vi "UI.vi"() -> ()   [LabVIEW 2016]
uses:
  interface_class/interface.lvclass
  <vilib>/Utility/miscctls.llb/LVPointTypeDef.ctl
  <vilib>/picture/picture.llb/imagedata.ctl
  MBinteractive_class/MBinteractive.lvclass
  tcp_work_class/tcp_work.lvclass
  serial_work_class/serial_work.lvclass
panel:
  in  "定时重发":T1={"重发日期"=enum."关闭", "重发时间"=enum."00点", "每周自动重发"=TRUE}
  in  "共享MN":bool
  out "剖面数据补发":bool
  out "日志信息补发":bool
  out "数据补发":bool
  in  "自动更新":bool
  in  "数据补传":bool caption="确定"
  out "与工控通信指示灯":bool
  in  "判断数据反馈":enum16{"非严格判断", "严格判断", "不判断"}(ring)
  in  "暂停上传":bool
  in  "配置表":bool caption="确定"
  in  "updateconfiguration":T2={"主机"="27.154.58.30", "用户"="update", "密码"="std23506", "远程路径"="数据传输系统\\平台数据传输系统.exe", "下载文件名"="平台数据传输系统.exe", "软件版本"=""}
  out "标题显示":string
  in  "更新":bool
  in  "系统编码选择框":string(combo)="地表水质量监测"
  in  "数据发送通道":enum16{"TCP", "VISA"}(ring)
  in  "baud rate":u32=9600 caption="波特率"
  in  "VISA resource name":refnum<visa-resource-name> caption="VISA资源名称"
  in  "实时数据发送时间间隔/min":i32=1
  in  "数据发送协议":enum16{"2005-212协议", "2017-212协议"}(ring)=enum."2017-212协议"
  in  "开机启动":bool
  in  "确定":bool
  in  "返回":bool
  in  "PW":string
  in  "MN":string
  in  "PORT":string
  in  "IP":string
  in  "站点设备":string
  in  "站点名称":string
  out "设置超时时间/min":i32=1
  out "状态信息":T3={"1st Error to Convert "=63, "步骤 "=enum."发送数据", "元素"="实时数据", "TCP服务端掉线计数"=0, "TCP掉线时间节点"="2019/05/08 15:24:17"} {"1st Error to Convert" items=["无错误", "参数错误", "内存已满", "超出区域", "文件结束", "文件已打开", "一般文件IO错误", "未找到文件", "文件权限错误", "磁盘已满", "路径副本", "打开过多文件", "未启用", "未找到资源文件", "无法添加资源", "未找到资源", "未找到图像", "图像内存错误", "画笔不存在", "配置错误类型", "配置未找到解析段", "配置解析错误", "配置内存错误", "错误外部代码格式", "错误外部代码偏移量", "外部代码不存在", "空窗口", "销毁窗口错误", "空菜单", "打印已中止", "错误打印记录", "打印驱动程序错误", "打印时窗口错误", "打印时内存错误", "打印对话框错误", "一般打印错误", "无效设备引用句柄", "设备未找到", "设备参数错误", "设备单位错误", "无法打开设备", "设备调用已中止", "一般错误", "用户已取消", "对象ID过低", "对象ID过高", "对象不在堆中", "未知的堆", "错误DefProc ID", "DefProc不在表格中", "范围外信息", "空方法", "未知信息", "不支持管理器调用", "错误地址", "连接过程中", "连接超时", "连接过程中", "不支持网络属性", "网络错误", "正在使用的地址", "系统缺少内存", "连接已中止", "连接已拒绝", "连接未建立", "连接已建立", "连接已关闭", "初始化错误（交互应用程序管理器）", "错误事件发生", "等待无约束事件发生处理程序", "事件发生队列溢出", "错误路径", "未发出信号量", "未识别类型（交互应用程序管理器）"]}
  out "数据接收超时指示灯":bool
  out "空闲时间/s":string
  out "系统时间":string
  out "实时小时数据上传":bool
  out "系统状态改变":bool
  out "软件版本":string
  out "掉线指示":bool
  out "核查数据上传":bool
  out "配置信息":T4
  in  "参数配置":bool
  out "反控数据发送":bool
  out "读取报文显示":string
  out "发送报文显示":string
  out "心跳包":bool
  out "通信状态":bool
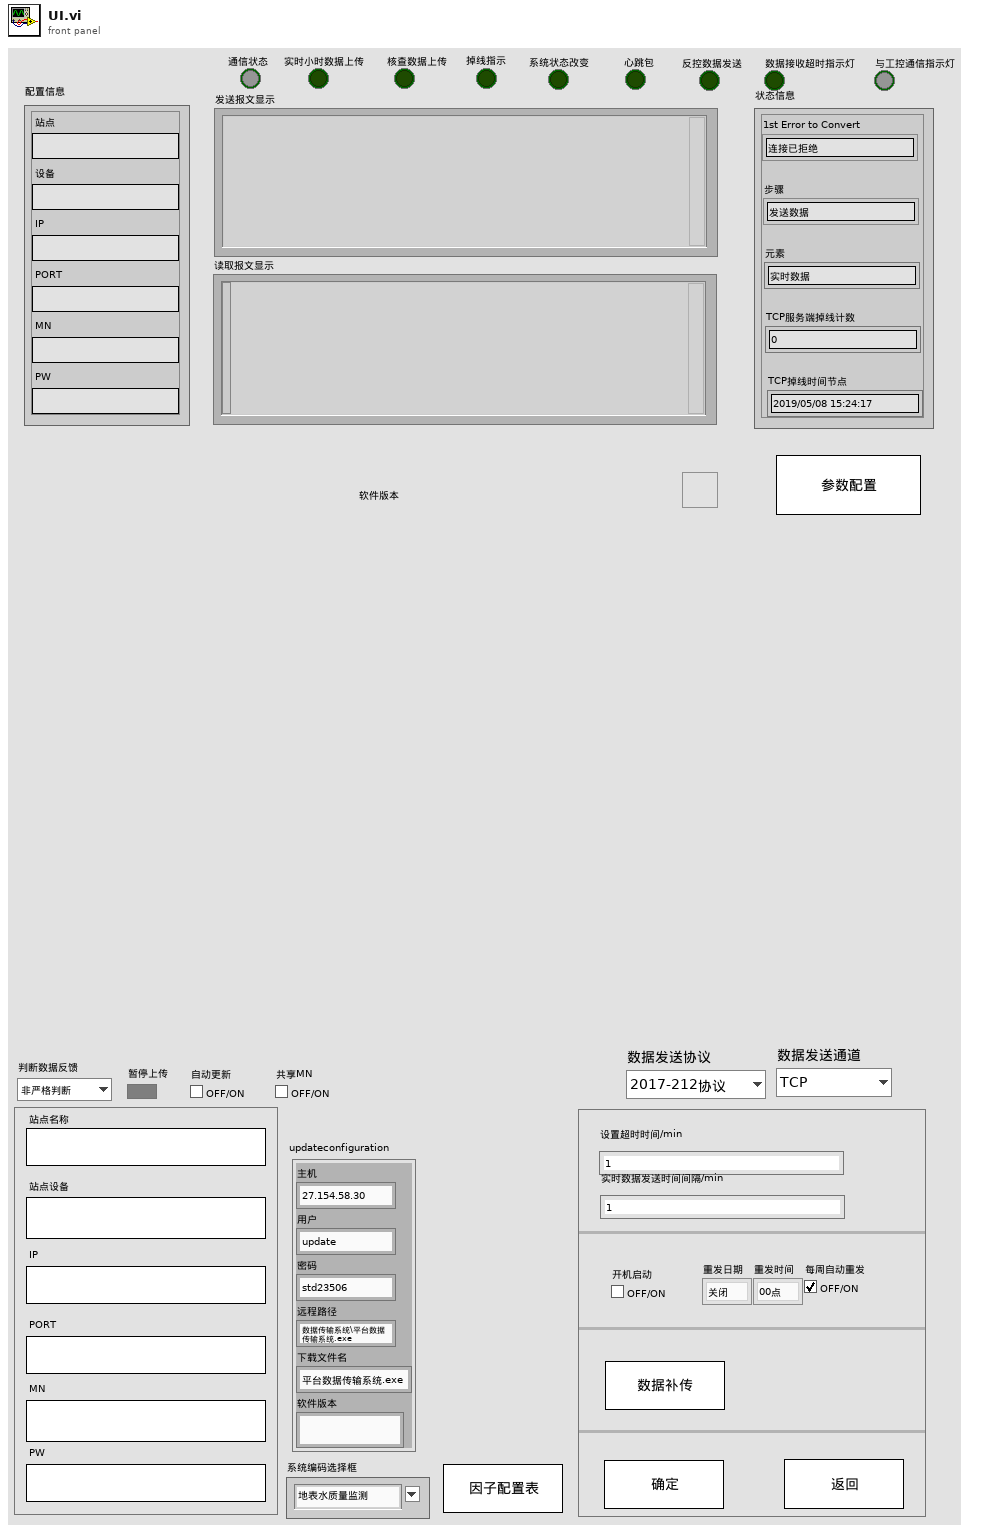
[diagram p1: front panel]
types:
  T1 = cluster{"重发日期":enum16{"关闭", "星期日", "星期一", "星期二", "星期三", "星期四", "星期五", "星期六"}, "重发时间":enum16{"00点", "01点", "02点", "03点", "04点", "05点", "06点", "07点", "08点", "09点", "10点", "11点", "12点", "13点", "14点", "15点", "16点", "17点", "18点", "19点", "20点", "21点", "22点", "23点"}, "每周自动重发":bool}
  T2 = cluster{"主机":string, "用户":string, "密码":string, "远程路径":string, "下载文件名":string, "软件版本":string}
  T3 = cluster{"1st Error to Convert ":i32, "步骤 ":enum16{"打开连接", "发送数据", "读取数据", "数据处理", "关闭连接"}, "元素":string, "TCP服务端掉线计数":i32, "TCP掉线时间节点":string}
  T4 = cluster{"站点":string, "设备":string, "IP":string, "PORT":string, "MN":string, "PW":string}
  T5 = typedef "imagedata.ctl" = cluster{"image type":i32, "image depth":i32, "image":u8[], "mask":u8[], "colors":u32[], "Rectangle":cluster{"left":i16, "top":i16, "right":i16, "bottom":i16}}
  T6 = typedef "LVPointTypeDef.ctl" = cluster{"Horizontal":i16, "Vertical":i16}
  T7 = cluster{"配置表格[0]":string, "配置表格[1]":string, "配置表格[2]":string, "配置表格[3]":string, "配置表格[4]":string, "配置表格[5]":string, "配置表格[6]":string, "配置表格[7]":string, "配置表格[8]":string, "配置表格[9]":string, "配置表格[10]":string, "配置表格[11]":string, "配置表格[12]":string, "配置表格[13]":string, "配置表格[14]":string, "配置表格[15]":string, "配置表格[16]":string, "配置表格[17]":string, "配置表格[18]":string, "配置表格[19]":string, "配置表格[20]":string, "配置表格[21]":string, "配置表格[22]":string, "配置表格[23]":string, "配置表格[24]":string, "配置表格[25]":string, "配置表格[26]":string, "配置表格[27]":string, "配置表格[28]":string, "配置表格[29]":string, "配置表格[30]":string, "配置表格[31]":string, "配置表格[32]":string, "配置表格[33]":string, "配置表格[34]":string, "配置表格[35]":string, "配置表格[36]":string}
  T8 = cluster{"[0]":dbl, "[1]":dbl, "[2]":dbl, "[3]":dbl, "[4]":dbl, "[5]":dbl, "[6]":dbl, "[7]":dbl, "[8]":dbl, "[9]":dbl, "[10]":dbl, "[11]":dbl, "[12]":dbl, "[13]":dbl, "[14]":dbl, "[15]":dbl, "[16]":dbl, "[17]":dbl, "[18]":dbl, "[19]":dbl, "[20]":dbl, "[21]":dbl, "[22]":dbl, "[23]":dbl, "[24]":dbl, "[25]":dbl, "[26]":dbl, "[27]":dbl, "[28]":dbl, "[29]":dbl, "[30]":dbl, "[31]":dbl, "[32]":dbl, "[33]":dbl, "[34]":dbl, "[35]":dbl, "[36]":dbl}
  T9 = cluster{"系统状态":bool, "运行模式":bool, "测量周期":bool, "超标留样":bool, "反控数据":bool, "核查数据上传":bool, "实时小时数据上传":bool, "数据接收超时指示灯":bool, "数据发送起始时间":timestamp, "与工控软件通信":bool, "发送报文首页显示":string, "读取报文首页显示":string, "掉线指示灯":bool, "TCP掉线时间节点":string}
  T10 = cluster{"updateconfiguration":cluster{"主机":string, "用户":string, "密码":string, "远程路径":string, "下载文件名":string, "软件版本":string}, "软件版本":string}
  T11 = cluster{"枚举":enum16{"打开连接", "发送数据", "读取数据", "数据处理", "关闭连接"}, "发送报文":string}
  T12 = cluster{"setini":string, "sysini":string, "hechaini":string, "actualwrite":string, "actualread":string, "datasent":string, "反控命令信息队列":string, "反控与仪器交互":string}
  T13 = cluster{"IP":string, "PORT":string, "VISA resource name":refnum<visa-resource-name>, "baud rate (9600)":u32, "data bits (8)":u16, "parity (0:none)":enum16{"None", "Odd", "Even", "Mark", "Space"}, "timeout (10sec)":u32}
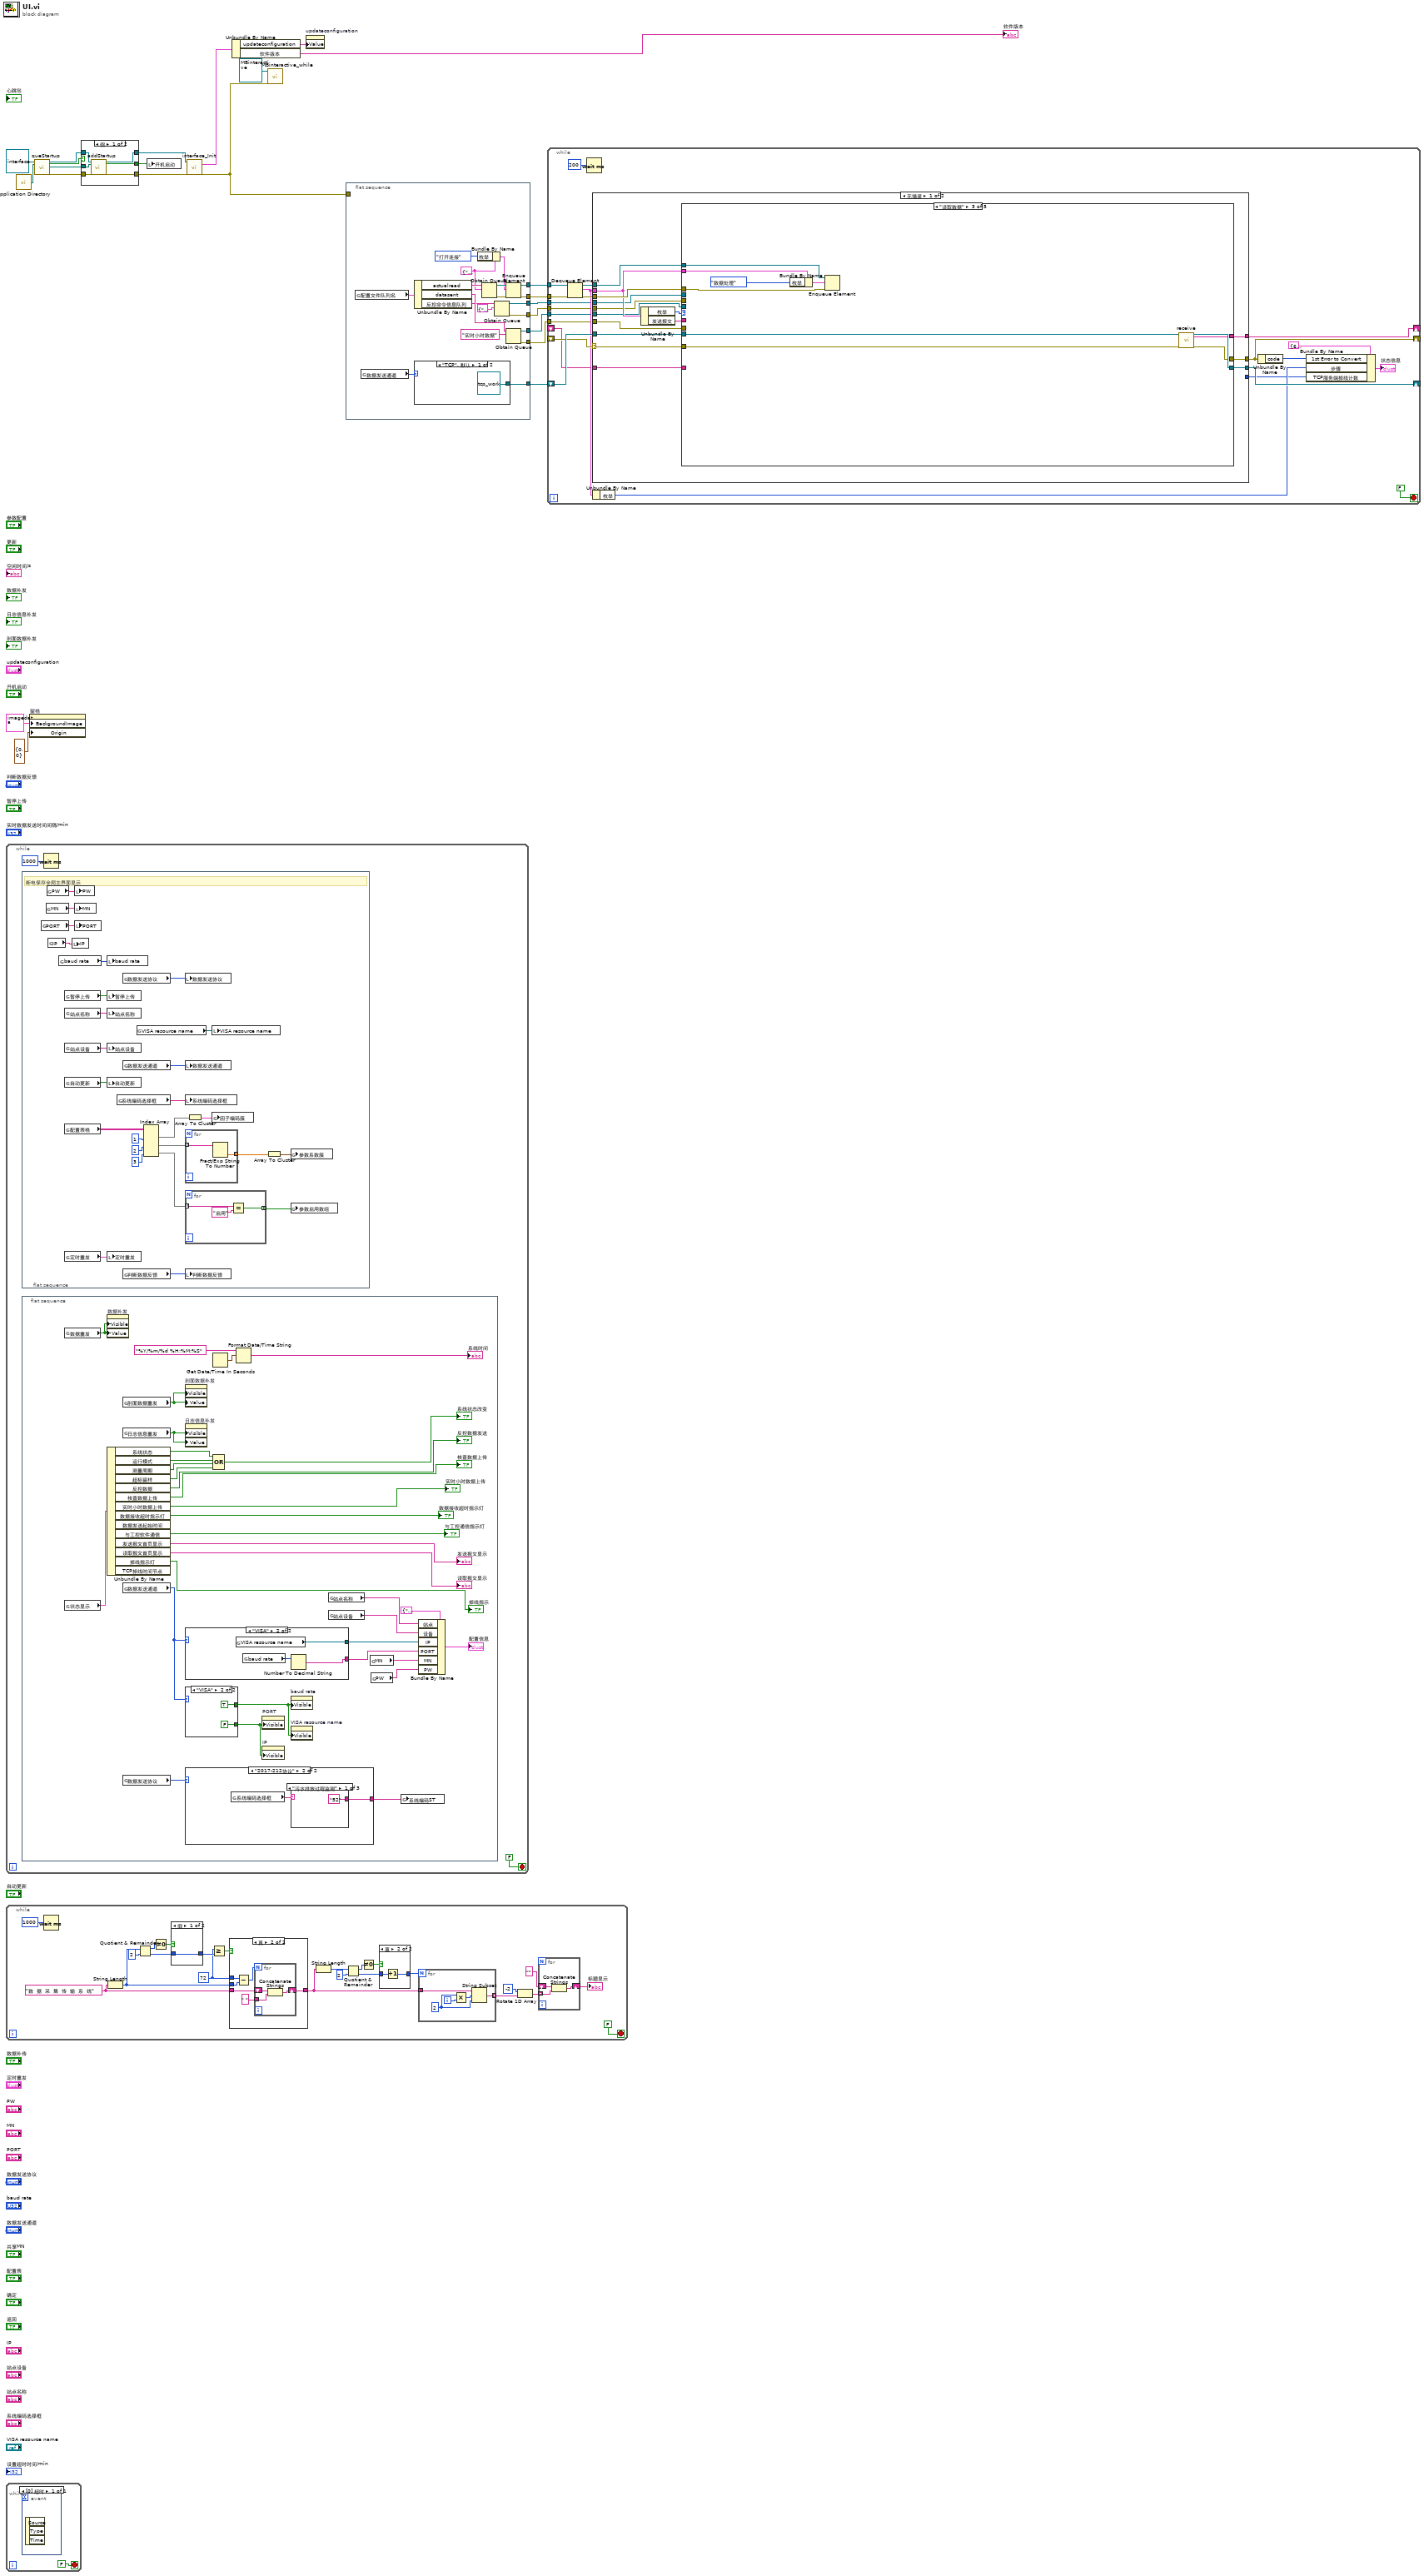
[diagram p0: block diagram]
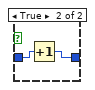
[diagram p3: hidden frame]
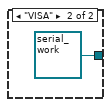
[diagram p5: hidden frame]
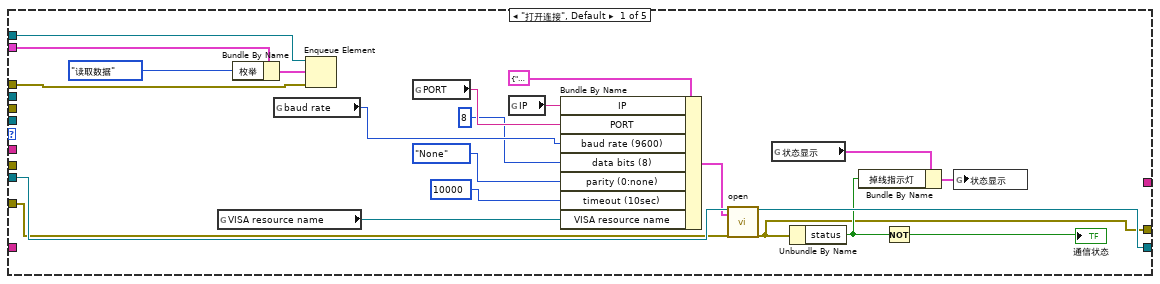
[diagram p6: hidden frame]
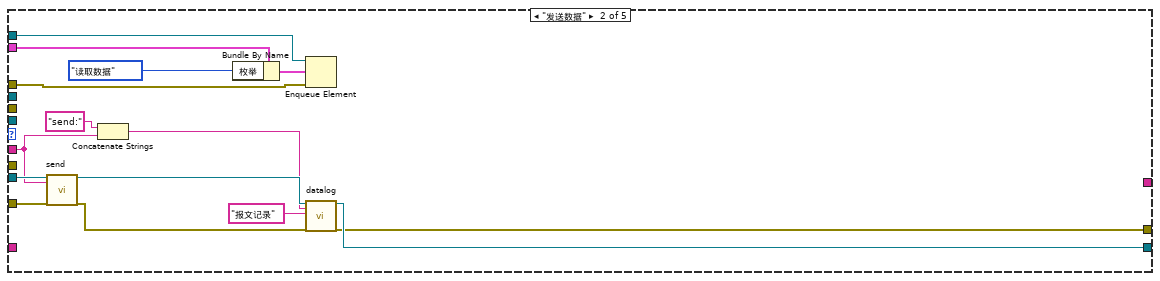
[diagram p7: hidden frame]
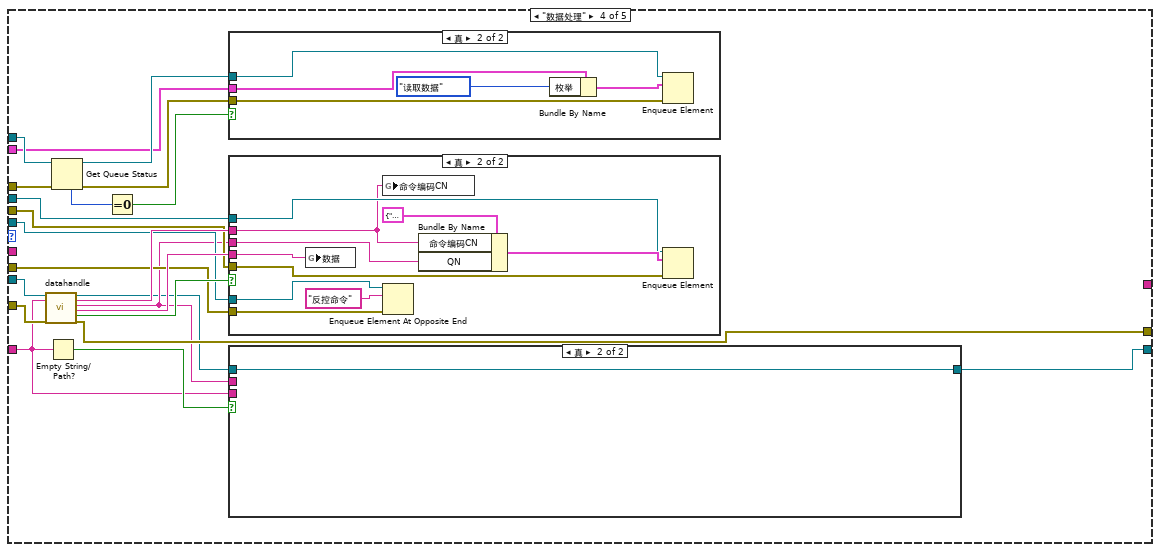
[diagram p8: hidden frame]
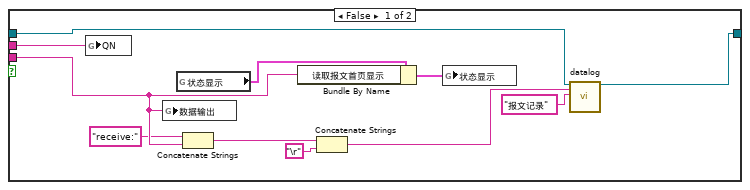
[diagram p9: hidden frame]
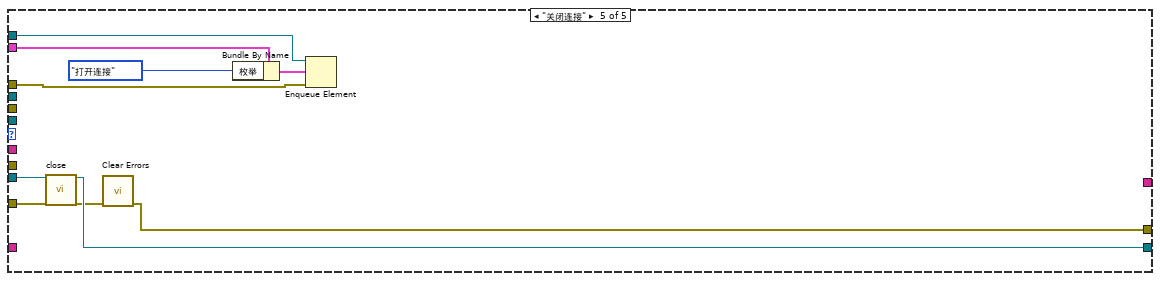
[diagram p12: hidden frame]
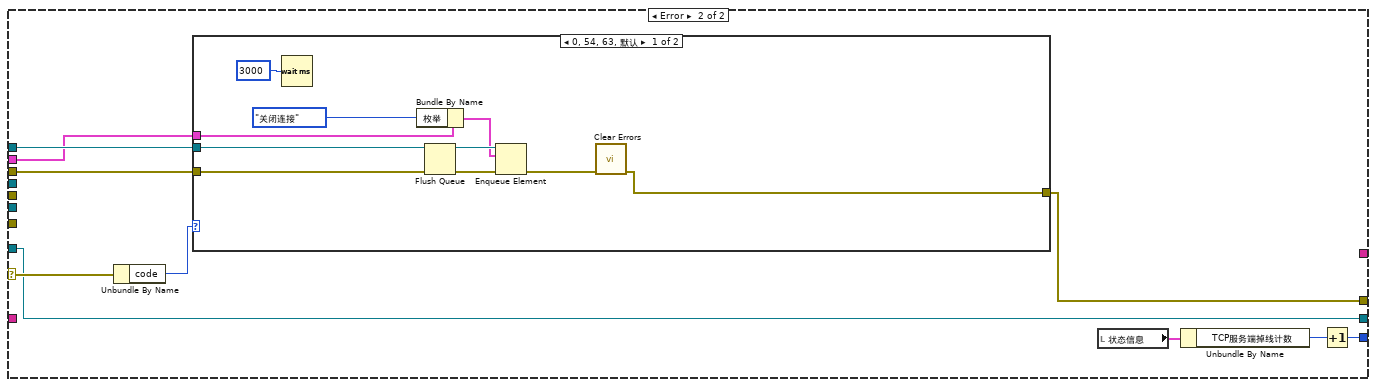
[diagram p13: hidden frame]
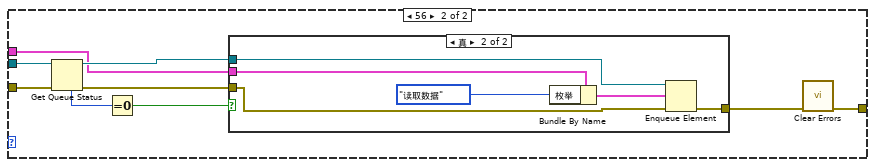
[diagram p14: hidden frame]
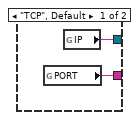
[diagram p16: hidden frame]
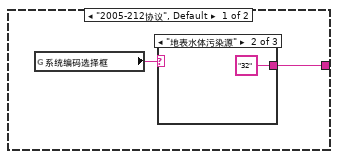
[diagram p17: hidden frame]
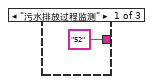
[diagram p18: hidden frame]
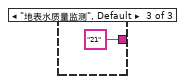
[diagram p19: hidden frame]
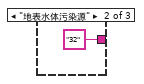
[diagram p20: hidden frame]
diagram:
  n1 = while {
    stop <- FALSE stop-if-true
    n2 = flat-sequence {
      frame #0 {
        # "断电保存全局主界面显示"
        n3 = global read "断电保存全局.vi" "PORT"() -> (w99:string)
        n4 = global read "断电保存全局.vi" "MN"() -> (w100:string)
        n5 = global read "断电保存全局.vi" "PW"() -> (w101:string)
        n6 = global read "断电保存全局.vi" "IP"() -> (w98:string)
        n7 = global read "断电保存全局.vi" "baud rate"() -> (w103:u32)
        n8 = global read "断电保存全局.vi" "暂停上传"() -> (w95:bool)
        n9 = global read "断电保存全局.vi" "站点名称"() -> (w96:string)
        n10 = global read "断电保存全局.vi" "站点设备"() -> (w97:string)
        n11 = global read "断电保存全局.vi" "自动更新"() -> (w94:bool)
        n12 = global read "断电保存全局.vi" "配置表格"() -> (w82:string[][])
        n13 = global read "断电保存全局.vi" "定时重发"() -> (w92:T1)
        n14 = local write "IP"(w98) -> ()
        n15 = local write "PW"(w101) -> ()
        n16 = local write "MN"(w100) -> ()
        n17 = local write "PORT"(w99) -> ()
        n18 = local write "baud rate"(w103) -> ()
        n19 = local write "暂停上传"(w95) -> ()
        n20 = local write "站点名称"(w96) -> ()
        n21 = local write "站点设备"(w97) -> ()
        n22 = local write "自动更新"(w94) -> ()
        n23 = local write "定时重发"(w92) -> ()
        n24 = global read "断电保存全局.vi" "系统编码选择框"() -> (w90:string)
        n25 = global read "断电保存全局.vi" "数据发送协议"() -> (w91:enum16{"2005-212协议", "2017-212协议"})
        n26 = global read "断电保存全局.vi" "数据发送通道"() -> (w78:enum16{"TCP", "VISA"})
        n27 = global read "断电保存全局.vi" "判断数据反馈"() -> (w93:enum16{"非严格判断", "严格判断", "不判断"})
        n28 = global read "断电保存全局.vi" "VISA resource name"() -> (w102:refnum<visa-resource-name>)
        n29 = Index Array(array=w82, index (col) #1=1 ("禁用的索引 (列)"), index (col) #2=2 ("索引 (列)"), index (col) #3=3 ("索引 (列)")) -> (element #1=w88:string[], element #2=w84:string[], element #3=w85:string[])  [unwired: 3 in]
        n30 = local write "数据发送协议"(w91) -> ()
        n31 = local write "数据发送通道"(w78) -> ()
        n32 = local write "系统编码选择框"(w90) -> ()
        n33 = for {
          tunnel: w84 -> [w105] mode=indexing
          tunnel: [w104] -> w83 mode=indexing
          n34 = Fract/Exp String To Number(string=w105) -> (number=w104:dbl)  [unwired: 3 in, 1 out]
        }
        n35 = for {
          tunnel: w85 -> [w108] mode=indexing
          tunnel: [w106] -> w79 mode=indexing
          n36 = Equal?(x=w108, y="启用") -> (x = y?=w106:bool)
        }
        n37 = local write "判断数据反馈"(w93) -> ()
        n38 = Array To Cluster(array=w88) -> (cluster=w80:T7)
        n39 = local write "VISA resource name"(w102) -> ()
        n40 = global write "断电保存全局.vi" "因子编码簇"(w80) -> ()
        n41 = Array To Cluster(array=w83) -> (cluster=w81:T8)
        n42 = global write "断电保存全局.vi" "参数系数簇"(w81) -> ()
        n43 = global write "断电保存全局.vi" "参数启用数组"(w79) -> ()
      }
    }
    n44 = flat-sequence {
      frame #0 {
        n45 = global read "断电保存全局.vi" "数据重发"() -> (w28:bool)
        n46 = global read "全局1.vi" "状态显示"() -> (w58:T9)
        n47 = property on="数据补发" class="Bool (严格)"("Visible"=w28, "Value"=w28) -> ()  [unwired: 2 in, 2 out]
        n48 = Unbundle By Name(w58) -> ("系统状态"=w57:bool, "运行模式"=w56:bool, "测量周期"=w55:bool, "超标留样"=w54:bool, "反控数据"=→"反控数据发送":bool, "核查数据上传"=→"核查数据上传":bool, "实时小时数据上传"=→"实时小时数据上传":bool, "数据接收超时指示灯"=→"数据接收超时指示灯":bool, "与工控软件通信"=→"与工控通信指示灯":bool, "发送报文首页显示"=→"发送报文显示":string, "读取报文首页显示"=→"读取报文显示":string, "掉线指示灯"=→"掉线指示":bool)  [unwired: 2 out]
        n49 = global read "断电保存全局.vi" "剖面数据重发"() -> (w26:bool)
        n50 = global read "断电保存全局.vi" "日志信息重发"() -> (w27:bool)
        n51 = global read "断电保存全局.vi" "数据发送通道"() -> (w33:enum16{"TCP", "VISA"})
        n52 = global read "断电保存全局.vi" "数据发送协议"() -> (w43:enum16{"2005-212协议", "2017-212协议"})
        n53 = property on="剖面数据补发" class="Bool (严格)"("Visible"=w26, "Value"=w26) -> ()  [unwired: 2 in, 2 out]
        n54 = property on="日志信息补发" class="Bool (严格)"("Visible"=w27, "Value"=w27) -> ()  [unwired: 2 in, 2 out]
        n55 = case shown="\"VISA\"" w33 {
          tunnel: [w60 w63] -> w37
          tunnel: [w59 w61] -> w36
          frame "TCP", Default {
            n56 = global read "断电保存全局.vi" "PORT"() -> (w59:string)
            n57 = global read "断电保存全局.vi" "IP"() -> (w60:string)
          }
          frame "VISA" {
            n58 = global read "断电保存全局.vi" "VISA resource name"() -> (w63:refnum<visa-resource-name>)
            n59 = global read "断电保存全局.vi" "baud rate"() -> (w62:u32)
            n60 = Number To Decimal String(number=w62) -> (decimal integer string=w61:string)  [unwired: 1 in]
          }
        }
        n61 = case shown="\"VISA\"" w33 {
          tunnel: [TRUE FALSE] -> w44
          tunnel: [FALSE TRUE] -> w45
          frame "TCP", Default {
          }
          frame "VISA" {
          }
        }
        n62 = case shown="\"2017-212协议\"" w43 {
          tunnel: [w64 w69] -> w42
          frame "2005-212协议", Default {
            n63 = global read "断电保存全局.vi" "系统编码选择框"() -> (w65:string)
            n64 = case shown="\"地表水体污染源\"" w65 {
              tunnel: ["52" ("设备编码MN") "32" ("设备编码MN") "21" ("设备编码MN")] -> w64
              frame "污水排放过程监测" {
              }
              frame "地表水体污染源" {
              }
              frame "地表水质量监测", Default {
              }
            }
          }
          frame "2017-212协议" {
            n65 = global read "断电保存全局.vi" "系统编码选择框"() -> (w70:string)
            n66 = case shown="\"污水排放过程监测\"" w70 {
              tunnel: ["52" ("设备编码MN") "32" ("设备编码MN") "21" ("设备编码MN")] -> w69
              frame "污水排放过程监测" {
              }
              frame "地表水体污染源" {
              }
              frame "地表水质量监测", Default {
              }
            }
          }
        }
        n67 = Get Date/Time In Seconds() -> (seconds since 1Jan1904=w30:timestamp)
        n68 = Compound Arithmetic op=OR ("复合运算")(w57, w56, w55, w54) -> (→"系统状态改变":bool)
        n69 = Format Date/Time String(time format string (%c)="%Y/%m/%d %H:%M:%S" ("时间格式字符串(%c)"), seconds (now)=w30) -> (date/time string=→"系统时间":string)  [unwired: 1 in]
        n70 = property on="PORT" class="Str"("Visible"=w44) -> ()  [unwired: 2 in, 2 out]
        n71 = property on="IP" class="Str"("Visible"=w44) -> ()  [unwired: 2 in, 2 out]
        n72 = property on="baud rate" class="DigNum (严格)"("Visible"=w45) -> ()  [unwired: 2 in, 2 out]
        n73 = property on="VISA resource name" class="VISAName"("Visible"=w45) -> ()  [unwired: 2 in, 2 out]
        n74 = global read "断电保存全局.vi" "站点名称"() -> (w39:string)
        n75 = global read "断电保存全局.vi" "站点设备"() -> (w38:string)
        n76 = global read "断电保存全局.vi" "MN"() -> (w35:string)
        n77 = global read "断电保存全局.vi" "PW"() -> (w34:string)
        n78 = global write "全局1.vi" "系统编码ST"(w42) -> ()
        n79 = Bundle By Name(cluster=T4 {"站点"="", "设备"="", "IP"="", "PORT"="", "MN"="", "PW"=""} ("配置信息"), "站点"=w39, "设备"=w38, "IP"=w37, "PORT"=w36, "MN"=w35, "PW"=w34) -> (→"配置信息":T4)
      }
    }
    n80 = Wait (ms)(milliseconds to wait=u32 1000 ("等待时间（毫秒）")) -> ()  [unwired: 1 out]
  }
  n81 = while {
    stop <- FALSE stop-if-true
    w111 = "数  据  采  集  传  输  系  统" ("标题显示")
    w112 = 72 ("字符框大小")
    n82 = Wait (ms)(milliseconds to wait=u32 1000 ("等待时间（毫秒）")) -> ()  [unwired: 1 out]
    n83 = String Length(string=w111) -> (length=w117:i32)
    n84 = Quotient & Remainder(x=w117, y=2) -> (x-y*floor(x/y)=w123:i32, floor(x/y)=w121:i32)
    n85 = Not Equal To 0?(x=w123) -> (x != 0?=w122:bool)
    n86 = case shown="假" w122 {
      tunnel: w121 -> [w145 w147]
      tunnel: [w145 w146] -> w119
      frame False {
      }
      frame True {
        n87 = Increment(x=w147) -> (x+1=w146:i32)
      }
    }
    n88 = Greater Or Equal?(x=w112, y=w119) -> (x >= y?=w120:bool)
    n89 = case shown="真" w120 {
      tunnel: w112 -> [_ w141]
      tunnel: w117 -> [_ w140]
      tunnel: w111 -> [w135 w137]
      tunnel: [w135 w136] -> w118
      frame False {
      }
      frame True {
        n90 = Subtract(x=w141, y=w140) -> (x-y=w139:i32)
        n91 = for {
          N: w139 -> [_]
          tunnel: " " ("字符串") -> [w144]
          shift-right: [w143] -> w136
          shift-left: w137 -> [w142]
          n92 = Concatenate Strings(w142, w144) -> (w143:string)
        }
      }
    }
    n93 = String Length(string=w118) -> (length=w130:i32)
    n94 = Quotient & Remainder(x=w130, y=2) -> (x-y*floor(x/y)=w128:i32, floor(x/y)=w126:i32)
    n95 = Not Equal To 0?(x=w128) -> (x != 0?=w127:bool)
    n96 = case shown="真" w127 {
      tunnel: w126 -> [w148 w150]
      tunnel: [w148 w149] -> w125
      frame False {
      }
      frame True {
        n97 = Increment(x=w150) -> (x+1=w149:i32)
      }
    }
    n98 = for {
      N: w125 -> [_]
      tunnel: w118 -> [w154]
      tunnel: [w155] -> w116 mode=indexing
      i -> [w153]
      w152 = 2 ("长度（剩余）")
      n99 = Multiply(x=w152, y=w153) -> (x*y=w151:i32)
      n100 = String Subset(string=w154, offset (0)=w151, length (rest)=w152) -> (substring=w155:string)
    }
    n101 = Rotate 1D Array(1:w116, 2:-2 ("n")) -> (0:w114:string[])
    n102 = for {
      tunnel: w114 -> [w134] mode=indexing
      shift-right: [w132] -> w110
      shift-left: "" -> [w133]
      n103 = Concatenate Strings(w133, w134) -> (w132:string)
    }
    "标题显示" <- w110
  }
  n104 = while {
    stop <- FALSE stop-if-true
    n105 = event shown="[0] 超时" {
      selector: _ -> [_]
      dyn-events: _ -> [_]
      timeout: _ -> [_]
      event Timeout {
        n106 = event-data() -> ()  [unwired: 1 in, 3 out]
      }
    }
  }
  n107 = call <vilib>:"Application Directory.vi"() -> ("Application Directory"=w22:path)
  n108 = property on="窗格" class="Pane"("BackgroundImage"=T5 {"image type"=0, "image depth"=24, "image"=array[12288000 elements], "mask"=[], "colors"=[], "Rectangle"={"left"=0, "top"=0, "right"=2560, "bottom"=1600}} ("image data"), "Origin"=T6 {"Horizontal"=0, "Vertical"=0} ("原点")) -> ()  [unwired: 2 in, 2 out]
  n109 = call-dynamic "queStartup.vi"("object in"=refnum<class "interface.lvclass"> refnum ("interface"), "启动文件路径"=w22) -> ("object out"=w20:refnum<class "interface.lvclass">, "包含启动项"=w21:bool, "启动文件路径"=w18:path, "error out"=w19:errorcluster)  [unwired: 14 in]
  n110 = case shown="假" w21 {
    selector: w21 -> [_ w165]
    tunnel: w20 -> [w162 w164]
    tunnel: w19 -> [w161 w163]
    tunnel: w18 -> [w160 _]
    tunnel: [w159 w165] -> w17
    tunnel: [w158 w164] -> w14
    tunnel: [w157 w163] -> w13
    frame False {
      n111 = call-dynamic "addStartup.vi"("object in"=w162, "启动文件路径"=w160, "error in (no error)"=w161) -> ("object out"=w158:refnum<class "interface.lvclass">, "添加成功标记"=w159:bool, "error out"=w157:errorcluster)  [unwired: 14 in]
    }
    frame True {
    }
  }
  n112 = local write "开机启动"(w17) -> ()
  n113 = call "interface_Init.vi"("object in"=w14, "error in (no error)"=w13) -> ("configout"=w12:T10, "error out"=w5:errorcluster)  [unwired: 15 in, 1 out]
  n114 = Unbundle By Name(w12) -> ("updateconfiguration"=w10:T2, "软件版本"=→"软件版本":string)
  n115 = call "MBinteractive_while.vi"("object in"=refnum<class "MBinteractive.lvclass"> refnum ("MBinteractive"), "error in (no error)"=w5) -> ()  [unwired: 16 in, 2 out]
  n116 = property on="updateconfiguration" class="Clust (严格)"("Value"=w10) -> ()  [unwired: 2 in, 2 out]
  n117 = flat-sequence {
    tunnel: [w177] -> w8
    tunnel: [w176] -> w7
    tunnel: [w175] -> w6
    tunnel: w5 -> [_]
    tunnel: [w169] -> w4
    tunnel: [w168] -> w3
    tunnel: [w167] -> w2
    tunnel: [w166] -> w1
    frame #0 {
      w179 = T11 {"枚举"=enum."打开连接", "发送报文"=""} ("data")
      n118 = global read "断电保存全局.vi" "配置文件队列名"() -> (w172:T12)
      n119 = global read "断电保存全局.vi" "数据发送通道"() -> (w184:enum16{"TCP", "VISA"})
      n120 = Unbundle By Name(w172) -> ("actualread"=w180:string, "datasent"=w171:string, "反控命令信息队列"=w170:string)
      n121 = case shown="\"TCP\", 默认" w184 {
        tunnel: [refnum<class "tcp_work.lvclass"> refnum ("tcp_work") refnum<class "serial_work.lvclass"> refnum ("serial_work")] -> w175
        frame "TCP", Default {
        }
        frame "VISA" {
        }
      }
      n122 = Bundle By Name(cluster=w179, "枚举"=enum16{"打开连接", "发送数据", "读取数据", "数据处理", "关闭连接"}."打开连接") -> (w181:T11)
      n123 = Obtain Queue(name (unnamed)=w180, element data type=w179) -> (queue out=w183:refnum<queue>, error out=w178:errorcluster)  [unwired: 3 in, 1 out]
      n124 = Obtain Queue(name (unnamed)=w170, element data type=cluster{"命令编码CN":string, "QN":string} {"命令编码CN"="", "QN"=""}) -> (queue out=w167:refnum<queue>, error out=w166:errorcluster)  [unwired: 3 in, 1 out]
      n125 = Enqueue Element(queue=w183, element=w181, error in (no error)=w178) -> (queue out=w177:refnum<queue>, error out=w176:errorcluster)  [unwired: 1 in, 1 out]
      n126 = Obtain Queue(name (unnamed)=w171, element data type="实时小时数据" ("元素")) -> (queue out=w169:refnum<queue>, error out=w168:errorcluster)  [unwired: 3 in, 1 out]
    }
  }
  n127 = while {
    tunnel: w8 -> [w208]
    tunnel: w7 -> [w207]
    shift-right: [w197] -> _
    shift-left: _ -> [w203]
    shift-right: [w204] -> _
    shift-left: w6 -> [w206]
    shift-right: [w192] -> _
    shift-left: _ -> [w191]
    tunnel: w4 -> [w190]
    tunnel: w3 -> [w189]
    tunnel: w2 -> [w188]
    tunnel: w1 -> [w187]
    stop <- FALSE stop-if-true
    n128 = Dequeue Element(queue=w208, error in (no error)=w207) -> (queue out=w198:refnum<queue>, element=w195:T11, error out=w199:errorcluster)  [unwired: 1 in, 1 out]
    n129 = Wait (ms)(milliseconds to wait=u32 200 ("等待时间（毫秒）")) -> ()  [unwired: 1 out]
    n130 = case shown="无错误" w203 {
      selector: w203 -> [w218 w339]
      tunnel: w195 -> [w215 w336]
      tunnel: w206 -> [w223 w333]
      tunnel: [w219 w334] -> w197
      tunnel: [w222 w333] -> w204
      tunnel: w199 -> [w217 w335]
      tunnel: w198 -> [w216 w337]
      tunnel: [_ w330] -> w193
      tunnel: [w209 _] -> w192
      tunnel: w191 -> [w214 _]
      tunnel: w190 -> [w213 _]
      tunnel: w189 -> [w212 _]
      tunnel: w188 -> [w211 _]
      tunnel: w187 -> [w210 _]
      frame No Error {
        n131 = Unbundle By Name(w215) -> ("枚举"=w221:enum16{"打开连接", "发送数据", "读取数据", "数据处理", "关闭连接"}, "发送报文"=w220:string)
        n132 = case shown="\"读取数据\"" w221 {
          tunnel: w223 -> [w245 w260 w270 w292 w329]
          tunnel: [w224 w249 w267 w290 w320] -> w219
          tunnel: [w244 w250 w268 w271 w327] -> w222
          tunnel: w220 -> [_ w247 _ _ _]
          tunnel: w218 -> [w234 w259 w269 w291 w328]
          tunnel: w217 -> [w229 w254 w262 w283 w325]
          tunnel: w216 -> [w231 w256 w264 w285 w323]
          tunnel: w215 -> [w230 w255 w263 w284 w321]
          tunnel: [_ _ w261 _ _] -> w209
          tunnel: w214 -> [_ _ _ w274 _]
          tunnel: w213 -> [_ _ _ w279 _]
          tunnel: w212 -> [_ _ _ w278 _]
          tunnel: w211 -> [_ _ _ w277 _]
          tunnel: w210 -> [_ _ _ w276 _]
          frame "打开连接", Default {
            n133 = global read "断电保存全局.vi" "VISA resource name"() -> (w236:refnum<visa-resource-name>)
            n134 = Bundle By Name(cluster=w230, "枚举"=enum16{"打开连接", "发送数据", "读取数据", "数据处理", "关闭连接"}."读取数据") -> (w232:T11)
            n135 = global read "断电保存全局.vi" "baud rate"() -> (w241:u32)
            n136 = Enqueue Element(queue=w231, element=w232, error in (no error)=w229) -> ()  [unwired: 1 in, 3 out]
            n137 = global read "断电保存全局.vi" "PORT"() -> (w242:string)
            n138 = global read "断电保存全局.vi" "IP"() -> (w243:string)
            n139 = Bundle By Name(cluster=T13 {"IP"="", "PORT"="", "VISA resource name"="", "baud rate (9600)"=115200, "data bits (8)"=8, "parity (0:none)"=enum."None", "timeout (10sec)"=10000} ("input"), "IP"=w243, "PORT"=w242, "baud rate (9600)"=w241, "data bits (8)"=u16 8, "parity (0:none)"=enum16{"None", "Odd", "Even", "Mark", "Space"}."None", "timeout (10sec)"=u32 10000, "VISA resource name"=w236) -> (w235:T13)
            n140 = call-dynamic "open.vi"("object in"=w245, "input"=w235, "error in (no error)"=w234) -> ("object out"=w244:refnum<class "tcp_work.lvclass">, "error out"=w224:errorcluster)  [unwired: 15 in]
            n141 = global read "全局1.vi" "状态显示"() -> (w228:T9)
            n142 = Unbundle By Name(w224) -> ("status"=w226:bool)
            n143 = Bundle By Name(cluster=w228, "掉线指示灯"=w226) -> (w227:T9)
            n144 = Not(x=w226) -> (.not. x?=→"通信状态":bool)
            n145 = global write "全局1.vi" "状态显示"(w227) -> ()
          }
          frame "发送数据" {
            n146 = call-dynamic "send.vi"("object in"=w260, "写入缓冲区"=w247, "error in (no error)"=w259) -> ("object out"=w253:refnum<class "tcp_work.lvclass">, "error out"=w251:errorcluster)  [unwired: 15 in]
            n147 = Concatenate Strings("send:" ("字符串"), w247) -> (w246:string)
            n148 = Bundle By Name(cluster=w255, "枚举"=enum16{"打开连接", "发送数据", "读取数据", "数据处理", "关闭连接"}."读取数据") -> (w257:T11)
            n149 = Enqueue Element(queue=w256, element=w257, error in (no error)=w254) -> ()  [unwired: 1 in, 3 out]
            n150 = call-dynamic "datalog.vi"("object in"=w253, "data"=w246, "filename"="报文记录", "error in (no error)"=w251) -> ("object out"=w250:refnum<class "tcp_work.lvclass">, "error out"=w249:errorcluster)  [unwired: 14 in]
          }
          frame "读取数据" {
            n151 = Bundle By Name(cluster=w263, "枚举"=enum16{"打开连接", "发送数据", "读取数据", "数据处理", "关闭连接"}."数据处理") -> (w265:T11)
            n152 = Enqueue Element(queue=w264, element=w265, error in (no error)=w262) -> ()  [unwired: 1 in, 3 out]
            n153 = call-dynamic "receive.vi"("object in"=w270, "error in (no error)"=w269) -> ("object out"=w268:refnum<class "tcp_work.lvclass">, "读取缓冲区"=w261:string, "error out"=w267:errorcluster)  [unwired: 14 in, 1 out]
          }
          frame "数据处理" {
            n154 = call-dynamic "datahandle.vi"("object in"=w292, "字符串"=w274, "error in (no error)"=w291) -> ("object out"=w272:refnum<class "tcp_work.lvclass">, "命令编码CN"=w281:string, "时间QN"=w273:string, "数据"=w280:string, "布尔"=w282:bool, "error out"=w290:errorcluster)  [unwired: 11 in]
            n155 = Empty String/Path?(string/path=w274) -> (empty?=w275:bool)
            n156 = Get Queue Status(queue=w285, error in (no error)=w283) -> (queue out=w287:refnum<queue>, error out=w286:errorcluster, # elements in queue=w289:i32)  [unwired: 1 in, 5 out]
            n157 = Equal To 0?(x=w289) -> (x = 0?=w288:bool)
            n158 = case shown="真" w288 {
              tunnel: w287 -> [_ w317]
              tunnel: w284 -> [_ w316]
              tunnel: w286 -> [_ w315]
              frame False {
              }
              frame True {
                n159 = Bundle By Name(cluster=w316, "枚举"=enum16{"打开连接", "发送数据", "读取数据", "数据处理", "关闭连接"}."读取数据") -> (w318:T11)
                n160 = Enqueue Element(queue=w317, element=w318, error in (no error)=w315) -> ()  [unwired: 1 in, 3 out]
              }
            }
            n161 = case shown="真" w282 {
              tunnel: w281 -> [_ w307]
              tunnel: w280 -> [_ w314]
              tunnel: w273 -> [_ w305]
              tunnel: w279 -> [_ w312]
              tunnel: w278 -> [_ w311]
              tunnel: w277 -> [_ w308]
              tunnel: w276 -> [_ w306]
              frame False {
              }
              frame True {
                n162 = global write "全局1.vi" "数据"(w314) -> ()
                n163 = global write "全局1.vi" "命令编码CN"(w307) -> ()
                n164 = Enqueue Element At Opposite End(queue=w312, element="反控命令" ("元素"), error in (no error)=w311) -> ()  [unwired: 1 in, 3 out]
                n165 = Bundle By Name(cluster=cluster{"命令编码CN":string, "QN":string} {"命令编码CN"="", "QN"=""}, "命令编码CN"=w307, "QN"=w305) -> (w309:cluster{"命令编码CN":string, "QN":string})
                n166 = Enqueue Element(queue=w308, element=w309, error in (no error)=w306) -> ()  [unwired: 1 in, 3 out]
              }
            }
            n167 = case shown="真" w275 {
              tunnel: w274 -> [w298 _]
              tunnel: w273 -> [w301 _]
              tunnel: w272 -> [w294 w304]
              tunnel: [w293 w304] -> w271
              frame False {
                n168 = global write "全局1.vi" "QN"(w301) -> ()
                n169 = global write "全局1.vi" "数据输出"(w298) -> ()
                n170 = global read "全局1.vi" "状态显示"() -> (w302:T9)
                n171 = Concatenate Strings("receive:" ("字符串"), w298) -> (w299:string)
                n172 = Bundle By Name(cluster=w302, "读取报文首页显示"=w298) -> (w303:T9)
                n173 = Concatenate Strings(w299, "\r") -> (w295:string)
                n174 = global write "全局1.vi" "状态显示"(w303) -> ()
                n175 = call-dynamic "datalog.vi"("object in"=w294, "data"=w295, "filename"="报文记录") -> ("object out"=w293:refnum<class "tcp_work.lvclass">)  [unwired: 15 in, 1 out]
              }
              frame True {
              }
            }
          }
          frame "关闭连接" {
            n176 = call-dynamic "close.vi"("object in"=w329, "error in (no error)"=w328) -> ("object out"=w327:refnum<class "tcp_work.lvclass">, "error out"=w326:errorcluster)  [unwired: 16 in]
            n177 = call <vilib>:"Clear Errors.vi"("error in (no error)"=w326) -> ("error out"=w320:errorcluster)  [unwired: 5 in, 1 out]
            n178 = Bundle By Name(cluster=w321, "枚举"=enum16{"打开连接", "发送数据", "读取数据", "数据处理", "关闭连接"}."打开连接") -> (w322:T11)
            n179 = Enqueue Element(queue=w323, element=w322, error in (no error)=w325) -> ()  [unwired: 1 in, 3 out]
          }
        }
      }
      frame Error {
        n180 = Unbundle By Name(w339) -> ("code"=w338:i32)
        n181 = case shown="0, 54, 63, 默认" w338 {
          tunnel: w337 -> [w345 w358]
          tunnel: w336 -> [w344 w353]
          tunnel: w335 -> [w343 w357]
          tunnel: [w341 w350] -> w334
          frame 0, 54, 63, Default {
            n182 = Wait (ms)(milliseconds to wait=u32 3000 ("等待时间（毫秒）")) -> ()  [unwired: 1 out]
            n183 = Bundle By Name(cluster=w344, "枚举"=enum16{"打开连接", "发送数据", "读取数据", "数据处理", "关闭连接"}."关闭连接") -> (w346:T11)
            n184 = Flush Queue(queue=w345, error in (no error)=w343) -> (queue out=w348:refnum<queue>, error out=w349:errorcluster)  [unwired: 1 out]
            n185 = Enqueue Element(queue=w348, element=w346, error in (no error)=w349) -> (error out=w342:errorcluster)  [unwired: 1 in, 2 out]
            n186 = call <vilib>:"Clear Errors.vi"("error in (no error)"=w342) -> ("error out"=w341:errorcluster)  [unwired: 5 in, 1 out]
          }
          frame 56 {
            n187 = Get Queue Status(queue=w358, error in (no error)=w357) -> (queue out=w355:refnum<queue>, error out=w354:errorcluster, # elements in queue=w356:i32)  [unwired: 1 in, 5 out]
            n188 = Equal To 0?(x=w356) -> (x = 0?=w352:bool)
            n189 = case shown="真" w352 {
              tunnel: w355 -> [_ w363]
              tunnel: w354 -> [w359 w362]
              tunnel: w353 -> [_ w361]
              tunnel: [w359 w360] -> w351
              frame False {
              }
              frame True {
                n190 = Bundle By Name(cluster=w361, "枚举"=enum16{"打开连接", "发送数据", "读取数据", "数据处理", "关闭连接"}."读取数据") -> (w364:T11)
                n191 = Enqueue Element(queue=w363, element=w364, error in (no error)=w362) -> (error out=w360:errorcluster)  [unwired: 1 in, 2 out]
              }
            }
            n192 = call <vilib>:"Clear Errors.vi"("error in (no error)"=w351) -> ("error out"=w350:errorcluster)  [unwired: 5 in, 1 out]
          }
        }
        n193 = local read "状态信息"() -> (w332:T3)
        n194 = Unbundle By Name(w332) -> ("TCP服务端掉线计数"=w331:i32)
        n195 = Increment(x=w331) -> (x+1=w330:i32)
      }
    }
    n196 = Unbundle By Name(w195) -> ("枚举"=w194:enum16{"打开连接", "发送数据", "读取数据", "数据处理", "关闭连接"})
    n197 = Unbundle By Name(w197) -> ("code"=w196:i32)
    n198 = Bundle By Name(cluster=T3 {"1st Error to Convert "=63, "步骤 "=enum."发送数据", "元素"="实时数据", "TCP服务端掉线计数"=0, "TCP掉线时间节点"="2019/05/08 15:24:17"} ("状态信息"), "1st Error to Convert"=w196, "步骤"=w194, "TCP服务端掉线计数"=w193) -> (→"状态信息":T3)
  }
